vi "SimulateAcquisition.vi"() -> ()   [LabVIEW 2015]
panel:
  out "x-y":u32
  out "filtered FFT":dbl[][](graph)
  out "FFT":dbl[][](graph)
  in  "stop":bool
  out "error out":errorcluster
  out "Intensity Graph":sgl[][](graph)
  in  "Tab Control":enum32{"file infos", "Page 2"}(tab)
  out "File Type":string
  out "Calibration":T1={"X Step"=1.0, "Y Step"=1.0, "Unit"=enum."Undefined"} {"Y Step" format="%.2f"; "X Step" format="%.2f"}
  out "loaded":T3(plugin-control)
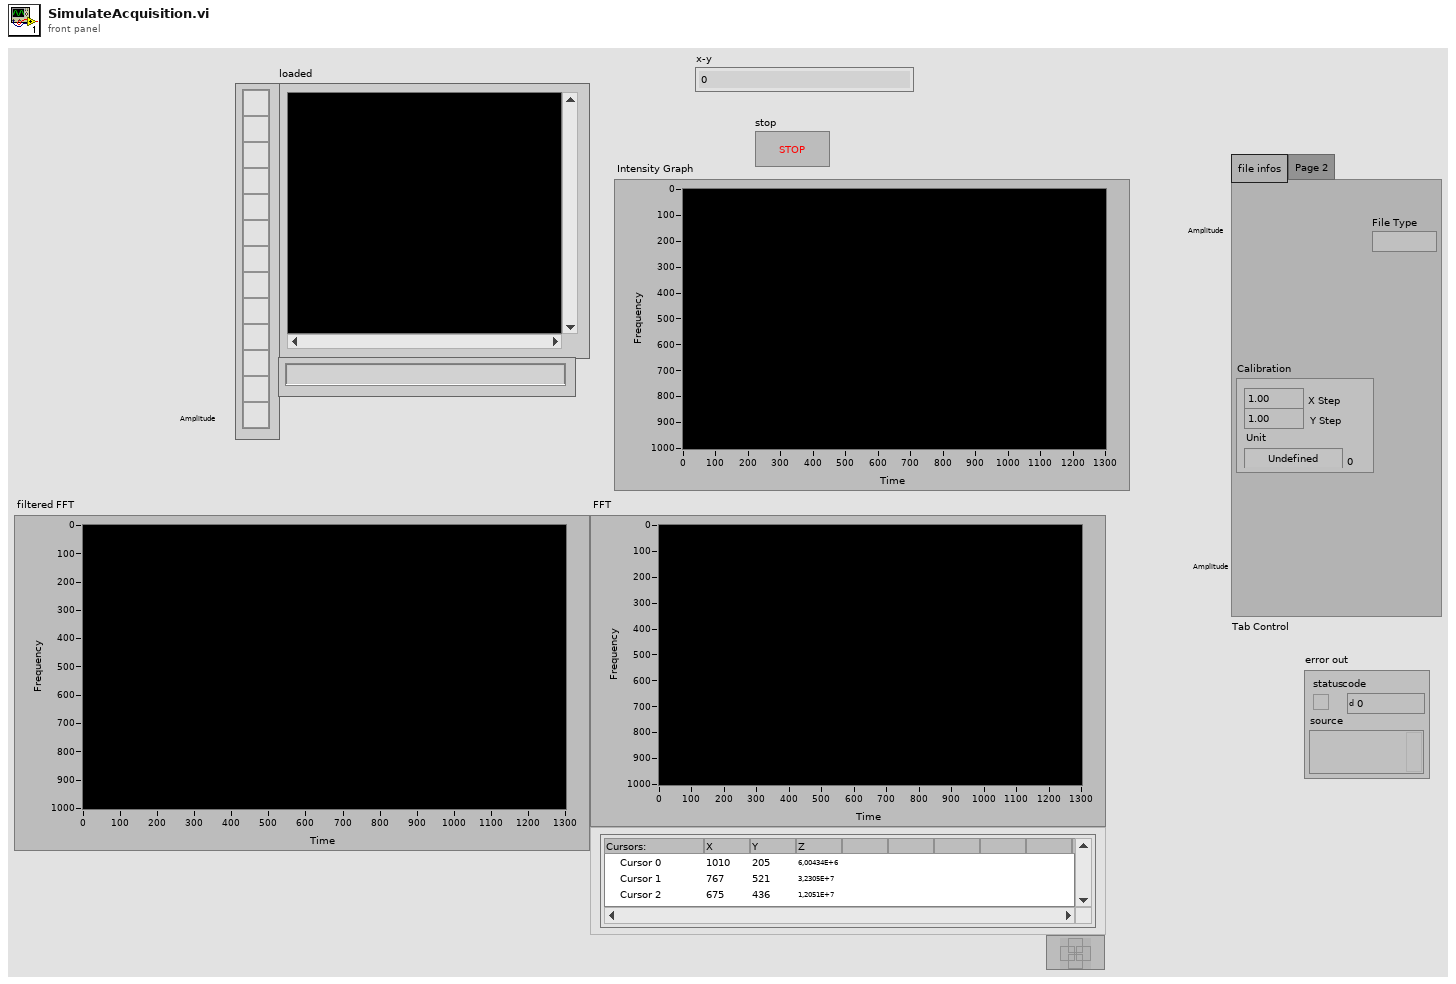
[diagram p1: front panel]
types:
  T1 = typedef "Simple Grid Descriptor" = cluster{"X Step":sgl, "Y Step":sgl, "Unit":T2}
  T2 = typedef "Image Unit" = enum32{"Undefined", "Angström", "Micrometer", "Millimeter", "Centimeter", "Meter", "Kilometer", "Microinch", "Inch", "Feet", "Nautical miles", "Standard miles", "Steps"}
  T3 = typedef "IMAQ Image.ctl" = refnum<image>
  T4 = typedef "Image Type" = u32
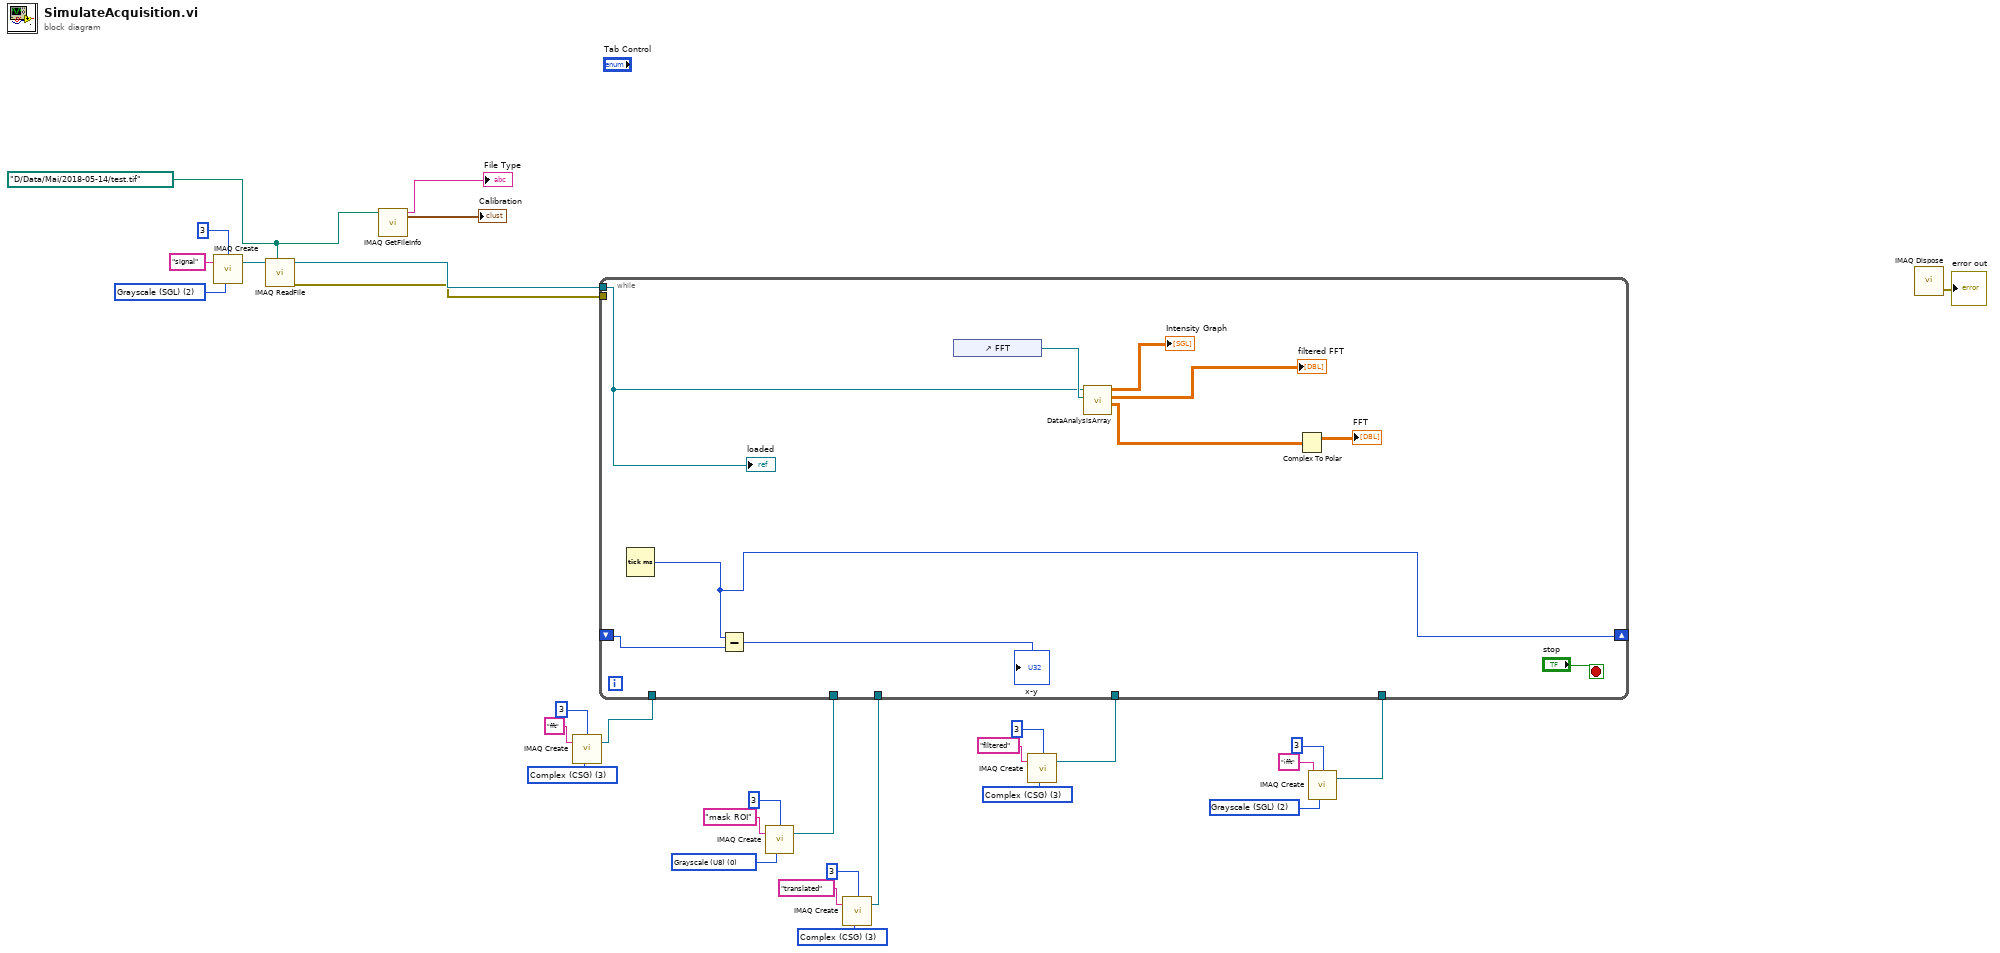
[diagram p0: block diagram]
diagram:
  w1 = T4 2 items=["Grayscale (U8)", "Grayscale (I16)", "Grayscale (SGL)", "Complex (CSG)", "RGB (U32)", "HSL (U32)", "RGB (U64)", "Grayscale (U16)"] ("Image Type")
  w5 = T4 3 items=["Grayscale (U8)", "Grayscale (I16)", "Grayscale (SGL)", "Complex (CSG)", "RGB (U32)", "HSL (U32)", "RGB (U64)", "Grayscale (U16)"] ("Image Type")
  w12 = T4 0 items=["Grayscale (U8)", "Grayscale (I16)", "Grayscale (SGL)", "Complex (CSG)", "RGB (U32)", "HSL (U32)", "RGB (U64)", "Grayscale (U16)"] ("Image Type")
  w16 = T4 3 items=["Grayscale (U8)", "Grayscale (I16)", "Grayscale (SGL)", "Complex (CSG)", "RGB (U32)", "HSL (U32)", "RGB (U64)", "Grayscale (U16)"] ("Image Type")
  w19 = T4 2 items=["Grayscale (U8)", "Grayscale (I16)", "Grayscale (SGL)", "Complex (CSG)", "RGB (U32)", "HSL (U32)", "RGB (U64)", "Grayscale (U16)"] ("Image Type")
  w22 = T4 3 items=["Grayscale (U8)", "Grayscale (I16)", "Grayscale (SGL)", "Complex (CSG)", "RGB (U32)", "HSL (U32)", "RGB (U64)", "Grayscale (U16)"] ("Image Type")
  w27 = path "D:/Data/Mai/2018-05-14/test.tif" ("File Path")
  n1 = call "IMAQ Create"("Border Size"=3, "Image Name"="signal", "Image Type"=w1) -> ("New Image"=w28:T3)  [unwired: 2 in, 1 out]
  n2 = call "IMAQ ReadFile"("File Path"=w27, "Image"=w28) -> ("error out"=w6:errorcluster, "Image Out"=w7:T3)  [unwired: 5 in, 3 out]
  n3 = call "IMAQ GetFileInfo"("File Path"=w27) -> ("File Type"=→"File Type":string, "Calibration"=→"Calibration":T1)  [unwired: 4 in, 5 out]
  n4 = call "IMAQ Create"("Border Size"=3, "Image Name"="fft", "Image Type"=w22) -> ("New Image"=w8:T3)  [unwired: 2 in, 1 out]
  n5 = call "IMAQ Create"("Border Size"=3, "Image Name"="mask ROI", "Image Type"=w12) -> ("New Image"=w9:T3)  [unwired: 2 in, 1 out]
  n6 = call "IMAQ Create"("Border Size"=3, "Image Name"="translated", "Image Type"=w5) -> ("New Image"=w2:T3)  [unwired: 2 in, 1 out]
  n7 = call "IMAQ Create"("Border Size"=3, "Image Name"="filtered", "Image Type"=w16) -> ("New Image"=w13:T3)  [unwired: 2 in, 1 out]
  n8 = call "IMAQ Create"("Border Size"=3, "Image Name"="ifft", "Image Type"=w19) -> ("New Image"=w17:T3)  [unwired: 2 in, 1 out]
  n9 = while {
    tunnel: w17 -> [_]
    tunnel: w13 -> [_]
    tunnel: w9 -> [_]
    tunnel: w8 -> [_]
    tunnel: w7 -> [w32]
    tunnel: w6 -> [_]
    tunnel: w2 -> [_]
    shift-right: [w37] -> _
    shift-left: _ -> [w38]
    stop <- "stop" stop-if-true
    n10 = Tick Count (ms)() -> (millisecond timer value=w37:u32)
    n11 = Subtract(x=w37, y=w38) -> (x-y=→"x-y":u32)
    n12 = control-ref of="FFT"() -> (w34:refnum<vi>)
    n13 = call "DataAnalysisArray.vi"("FFT 2"=w34, "Image IN"=w32) -> ("FFT {X}"=w36:cdb[][], "filtered FFT"=→"filtered FFT":cdb[][], "Image Pixels (Float)"=→"Intensity Graph":sgl[][])  [unwired: 5 in, 2 out]
    n14 = Complex To Polar(r * e^(i*theta)=w36) -> (r=→"FFT":dbl[][])  [unwired: 1 out]
    "loaded" <- w32
  }
  n15 = call "IMAQ Dispose"() -> ("error out"=→"error out":errorcluster)  [unwired: 6 in]
